vi "Estados_FGV.vi"(0 "Estados_IN":bool[](array[boolean]), 4 "Opción":enum16{"Write", "Read"}(ring), 5 "Error In":errorcluster) -> (14 "Estados_OUT":bool[](array[boolean]), 19 "Error Out":errorcluster)   [LabVIEW 2013]
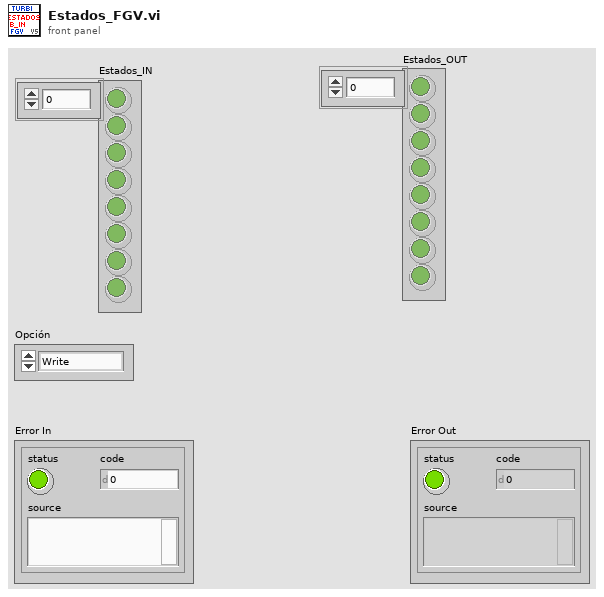
[diagram p1: front panel]
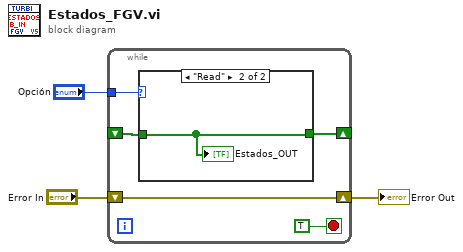
[diagram p0: block diagram]
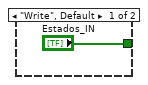
[diagram p2: hidden frame]
diagram:
  n1 = while {
    shift-right: [w7] -> w2
    shift-left: "Error In" -> [w7]
    tunnel: "Opción" -> [w6]
    shift-right: [w5] -> _
    shift-left: _ -> [w4]
    stop <- TRUE stop-if-true
    n2 = case shown="\"Read\"" w6 {
      tunnel: ["Estados_IN" w10] -> w5
      tunnel: w4 -> [_ w10]
      frame "Write", Default {
      }
      frame "Read" {
        "Estados_OUT" <- w10
      }
    }
  }
  "Error Out" <- w2
